vi "Proyecto.vi"() -> ()   [LabVIEW 2018]
uses:
  <vilib>/addons/Wavelet Analysis/application.llb/WA Detrend (Waveform).vi
  <vilib>/addons/Wavelet Analysis/application.llb/WA Multiscale Peak Detection (Waveform).vi
  <vilib>/addons/_Advanced Signal Processing/NI_AdvSigProcWA.lvlib
panel:
  out "Señal ECG filtrada":dynamicdata(graph)
  in  "stop":bool
  out "Trend Removed Signal":waveform(dbl)(graph)
  in  "threshold":dbl format="%#_13g"
  out "XY Graph":cluster{"Y":dbl[], "Y":dbl[]}[](graph)
  out "Nise Removed Signal":waveform(dbl)(graph)
  out "Mean (DC)":dbl
  out "Negative Peak":dbl
  out "Peak to Peak":dbl
  out "Positive Peak":dbl
  out "Señal ECG sin filtrar":dynamicdata(graph)
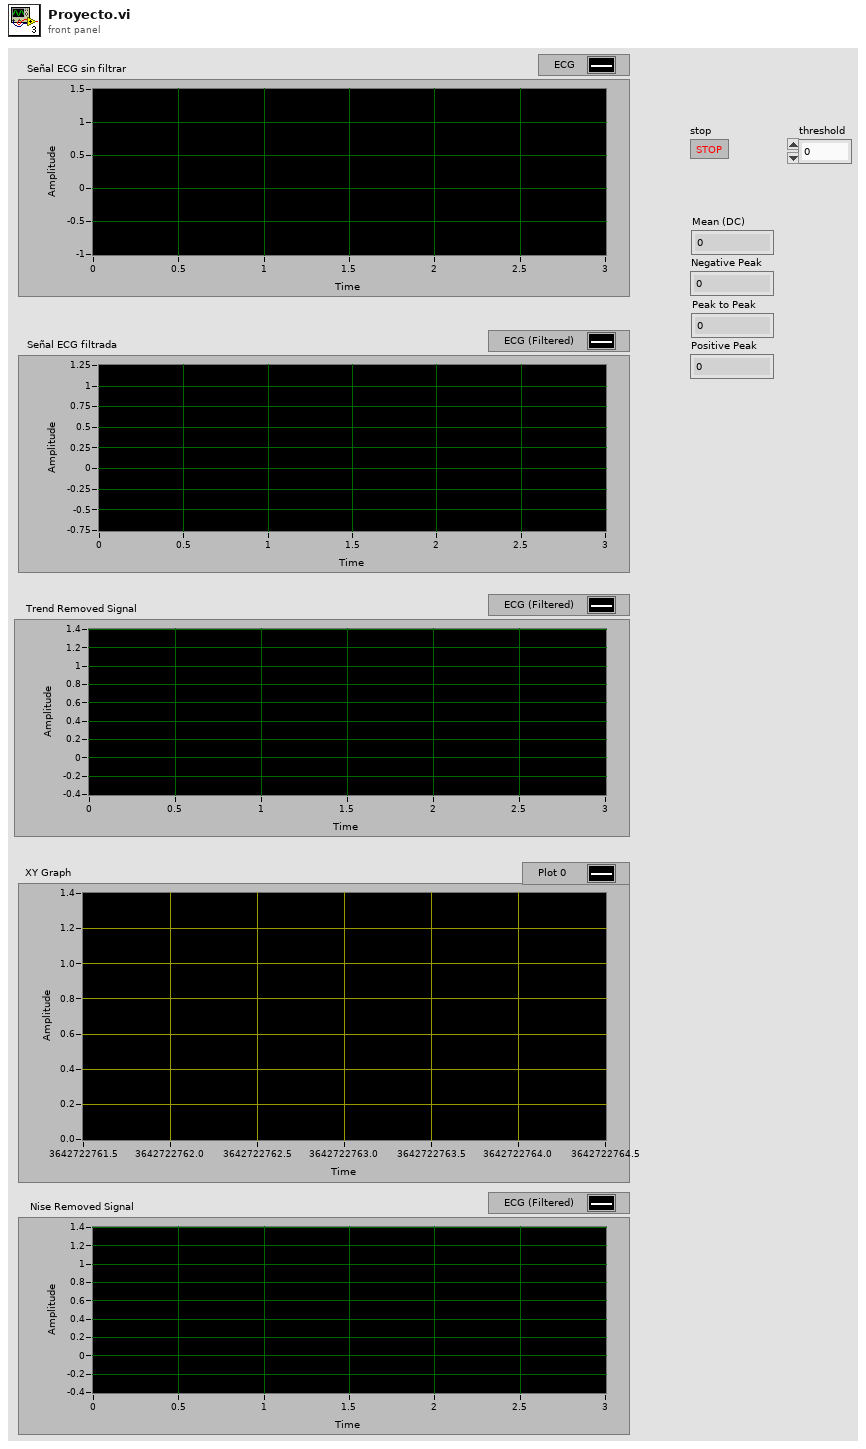
[diagram p1: front panel]
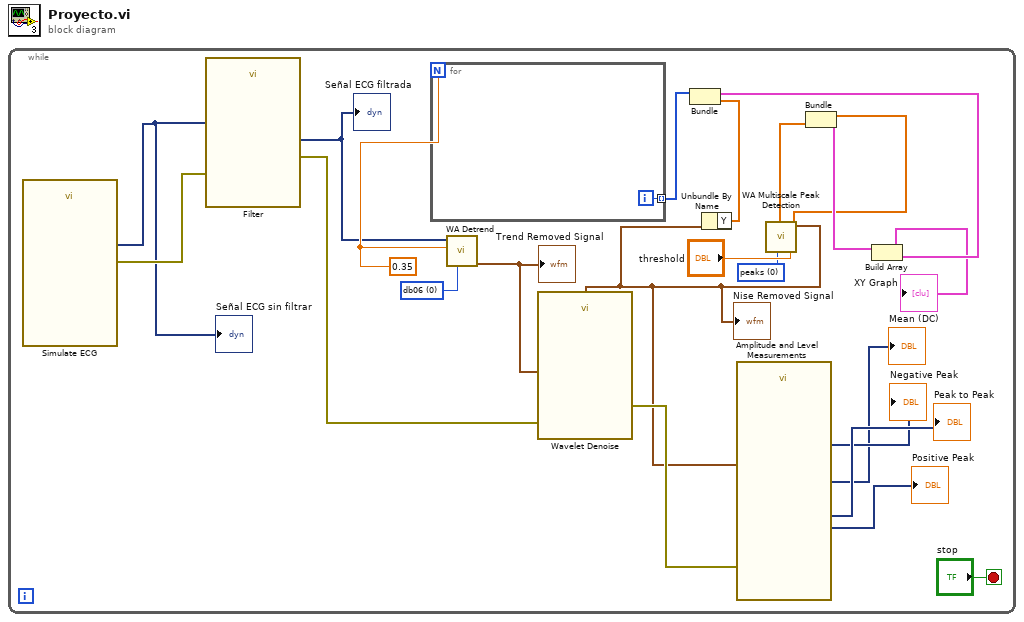
[diagram p0: block diagram]
diagram:
  n1 = while {
    stop <- "stop" stop-if-true
    w13 = u16 0 items=["db06"=0, "db03"=1, "db04"=2, "db05"=3, "db06"=4, "db07"=5, "db08"=6, "db09"=7, "db10"=8, "db11"=9, "db12"=10, "db13"=11, "db14"=12, "Haar"=13, "bior1_3"=14, "bior1_5"=15, "bior2_2"=16, "bior2_4"=17, "bior2_6"=18, "bior2_8"=19, "bior3_1"=20, "bior3_3"=21, "bior3_5"=22, "bior3_7"=23, "bior3_9"=24, "bior4_4 (FBI)"=25, "bior5_5"=38, "bior6_8"=39, "coif1"=26, "coif2"=27, "coif3"=28, "coif4"=29, "coif5"=30, "sym2"=31, "sym3"=32, "sym4"=33, "sym5"=34, "sym6"=35, "sym7"=36, "sym8"=37] ("wavelet")
    w5 = u16 0 items=["peaks", "valleys"] ("peaks/valleys")
    w14 = 0.35 ("threshold frequency")
    n2 = call "Simulate ECG"() -> ("error out"=w2:errorcluster, "ECG"=w1:dynamicdata)  [unwired: 10 in]
    "Señal ECG sin filtrar" <- w1
    n3 = call "Filter"("error in (no error)"=w2, "Signal"=w1) -> ("error out"=w12:errorcluster, "Filtered Signal"=w4:dynamicdata)  [unwired: 8 in]
    "Señal ECG filtrada" <- w4
    n4 = for {
      N: w14 -> [_]
      tunnel: [w24] -> w20 mode=indexing
      i -> [w24]
    }
    n5 = call-poly <vilib>:"WA Detrend.vi"("wavelet"=w13, "threshold frequency"=w14, "signal"=w4) -> ("detrended signal"=w3:waveform(dbl))  [unwired: 6 in, 2 out]
    "Trend Removed Signal" <- w3
    n6 = call "Wavelet Denoise"("error in (no error)"=w12, "Signal"=w3) -> ("error out"=w7:errorcluster, "Denoised Signal"=w6:waveform(dbl))  [unwired: 8 in]
    "Nise Removed Signal" <- w6
    n7 = Unbundle By Name(w6) -> ("Y"=w21:dbl[])
    n8 = Bundle(w20, "Y"=w21) -> (w22:cluster{i32[], "Y":dbl[]})  [unwired: 1 in]
    n9 = call "Amplitude and Level Measurements"("Signals"=w6, "error in (no error)"=w7) -> ("Mean (DC)"=→"Mean (DC)":dynamicdata, "Negative Peak"=→"Negative Peak":dynamicdata, "Positive Peak"=→"Positive Peak":dynamicdata, "Peak to Peak"=→"Peak to Peak":dynamicdata)  [unwired: 9 in, 1 out]
    n10 = call-poly <vilib>:"WA Multiscale Peak Detection.vi"("peaks/valleys"=w5, "threshold"="threshold", "signal"=w6) -> ("amplitude"=w17:dbl[], "location"=w16:dbl[])  [unwired: 4 in, 3 out]
    n11 = Bundle("location"=w16, "amplitude"=w17) -> (w18:cluster{"location":dbl[], "amplitude":dbl[]})  [unwired: 1 in]
    n12 = Build Array(w18, w22) -> (→"XY Graph":cluster{"location":dbl[], "Y":dbl[]}[])
  }
